vi "main(Test DQMH modules).bak.vi"() -> ()   [LabVIEW 2018, in "Application.lvlib"] (continued)
            n2019 = Select(t="Quece timeout", s=w4663, f=w4660) -> (s? t:f=w4659:string)
            n2020 = call "string log (SubVI).vi"("Enum"=enum16{"Init", "Log", "Read"}."Log", "state Name"=w4659) -> ()  [unwired: 8 in, 2 out]
          }
          frame condition #1 {
          }
        }
        n2021 = call "progress string(SubVI).vi"("String 3"=w4625, "String in"=w4626) -> ("String out"=w4627:string)  [unwired: 9 in]
        n2022 = call "FGV Driver Data.vi"("DUT index(1-60)"=w4624) -> ("DUT SC"=w4623:bool)  [unwired: 7 in, 3 out]
        n2023 = case shown="False" w4623 {
          tunnel: [w4652 _] -> w4632
          tunnel: w4629 -> [w4651 _]
          frame False {
            w4639 = T11 {"command"="", "command data"=variant} ("element")
            w4638 = "MEAS.mux6_1"
            n2024 = To Variant(anything=T4."mux6-1_channel0" ("mux6_1(3wires)_encode")) -> (Variant=w4637:variant)
            n2025 = To Variant(anything=T4."mux6_1_channel5_3" ("mux6_1(3wires)_encode")) -> (Variant=w4649:variant)
            n2026 = To Variant(anything=T4."mux6_1_channel5_2" ("mux6_1(3wires)_encode")) -> (Variant=w4647:variant)
            n2027 = Bundle By Name(cluster=w4639, "command"=w4638, "command data"=w4647) -> (w4646:T11)
            n2028 = Bundle By Name(cluster=w4639, "command"=w4638, "command data"=w4649) -> (w4645:T11)
            n2029 = Bundle By Name(cluster=w4639, "command"=w4638, "command data"=w4637) -> ()  [unwired: 1 out]
            n2030 = Bundle By Name(cluster=w4639, "command"="MEAS.DMM dual read") -> (w4643:T11)
            n2031 = Build Array(w4646, w4645, w4643) -> (w4641:T11[])
            n2032 = Reverse 1D Array(array=w4641) -> (reversed array=w4642:T11[])
            n2033 = for {
              tunnel: [w4658] -> w4652 mode=indexing
              tunnel: w4651 -> [w4657]
              tunnel: w4642 -> [w4656] mode=indexing
              n2034 = Unbundle By Name(w4656) -> ("command"=w4655:string, "command data"=w4654:variant)
              n2035 = call "App enquece.vi"("Priority Enquece"=TRUE, "command data"=w4654, "command"=w4655, "queue in"=w4657) -> ("error out"=w4658:errorcluster)  [unwired: 6 in, 1 out]
            }
          }
          frame True {
          }
        }
        n2036 = Merge Errors(w4630, w4632) -> (w4631:errorcluster)
      }
      frame "Test DRV 36" {
        w4665 = 36  # DUT index(0-59)
        n2037 = disable-structure shown="LOGGING==TRUE" {
          disable-tunnel: w4666 -> [w4701 _]
          frame condition #0 (active) {
            n2038 = Empty String/Path?(string/path=w4701) -> (empty?=w4704:bool)
            n2039 = Select(t="Quece timeout", s=w4704, f=w4701) -> (s? t:f=w4700:string)
            n2040 = call "string log (SubVI).vi"("Enum"=enum16{"Init", "Log", "Read"}."Log", "state Name"=w4700) -> ()  [unwired: 8 in, 2 out]
          }
          frame condition #1 {
          }
        }
        n2041 = call "progress string(SubVI).vi"("String 3"=w4666, "String in"=w4667) -> ("String out"=w4668:string)  [unwired: 9 in]
        n2042 = call "FGV Driver Data.vi"("DUT index(1-60)"=w4665) -> ("DUT SC"=w4664:bool)  [unwired: 7 in, 3 out]
        n2043 = case shown="False" w4664 {
          tunnel: [w4693 _] -> w4673
          tunnel: w4670 -> [w4692 _]
          frame False {
            w4680 = T11 {"command"="", "command data"=variant} ("element")
            w4679 = "MEAS.mux6_1"
            n2044 = To Variant(anything=T4."mux6-1_channel0" ("mux6_1(3wires)_encode")) -> (Variant=w4678:variant)
            n2045 = To Variant(anything=T4."mux6_1_channel6_3" ("mux6_1(3wires)_encode")) -> (Variant=w4690:variant)
            n2046 = To Variant(anything=T4."mux6_1_channel6_2" ("mux6_1(3wires)_encode")) -> (Variant=w4688:variant)
            n2047 = Bundle By Name(cluster=w4680, "command"=w4679, "command data"=w4688) -> (w4687:T11)
            n2048 = Bundle By Name(cluster=w4680, "command"=w4679, "command data"=w4690) -> (w4686:T11)
            n2049 = Bundle By Name(cluster=w4680, "command"=w4679, "command data"=w4678) -> ()  [unwired: 1 out]
            n2050 = Bundle By Name(cluster=w4680, "command"="MEAS.DMM dual read") -> (w4684:T11)
            n2051 = Build Array(w4687, w4686, w4684) -> (w4682:T11[])
            n2052 = Reverse 1D Array(array=w4682) -> (reversed array=w4683:T11[])
            n2053 = for {
              tunnel: [w4699] -> w4693 mode=indexing
              tunnel: w4692 -> [w4698]
              tunnel: w4683 -> [w4697] mode=indexing
              n2054 = Unbundle By Name(w4697) -> ("command"=w4696:string, "command data"=w4695:variant)
              n2055 = call "App enquece.vi"("Priority Enquece"=TRUE, "command data"=w4695, "command"=w4696, "queue in"=w4698) -> ("error out"=w4699:errorcluster)  [unwired: 6 in, 1 out]
            }
          }
          frame True {
          }
        }
        n2056 = Merge Errors(w4671, w4673) -> (w4672:errorcluster)
      }
      frame "Test DRV 37" {
        w4706 = 37  # DUT index(0-59)
        n2057 = disable-structure shown="LOGGING==TRUE" {
          disable-tunnel: w4707 -> [w4742 _]
          frame condition #0 (active) {
            n2058 = Empty String/Path?(string/path=w4742) -> (empty?=w4745:bool)
            n2059 = Select(t="Quece timeout", s=w4745, f=w4742) -> (s? t:f=w4741:string)
            n2060 = call "string log (SubVI).vi"("Enum"=enum16{"Init", "Log", "Read"}."Log", "state Name"=w4741) -> ()  [unwired: 8 in, 2 out]
          }
          frame condition #1 {
          }
        }
        n2061 = call "progress string(SubVI).vi"("String 3"=w4707, "String in"=w4708) -> ("String out"=w4709:string)  [unwired: 9 in]
        n2062 = call "FGV Driver Data.vi"("DUT index(1-60)"=w4706) -> ("DUT SC"=w4705:bool)  [unwired: 7 in, 3 out]
        n2063 = case shown="False" w4705 {
          tunnel: [w4734 _] -> w4714
          tunnel: w4711 -> [w4733 _]
          frame False {
            w4721 = T11 {"command"="", "command data"=variant} ("element")
            w4720 = "MEAS.mux6_1"
            n2064 = To Variant(anything=T4."mux6-1_channel0" ("mux6_1(3wires)_encode")) -> (Variant=w4719:variant)
            n2065 = To Variant(anything=T4."mux6_1_channel1_3" ("mux6_1(3wires)_encode")) -> (Variant=w4731:variant)
            n2066 = To Variant(anything=T4."mux6-1_channel1_2" ("mux6_1(3wires)_encode")) -> (Variant=w4729:variant)
            n2067 = Bundle By Name(cluster=w4721, "command"=w4720, "command data"=w4729) -> (w4728:T11)
            n2068 = Bundle By Name(cluster=w4721, "command"=w4720, "command data"=w4731) -> (w4727:T11)
            n2069 = Bundle By Name(cluster=w4721, "command"=w4720, "command data"=w4719) -> ()  [unwired: 1 out]
            n2070 = Bundle By Name(cluster=w4721, "command"="MEAS.DMM dual read") -> (w4725:T11)
            n2071 = Build Array(w4728, w4727, w4725) -> (w4723:T11[])
            n2072 = Reverse 1D Array(array=w4723) -> (reversed array=w4724:T11[])
            n2073 = for {
              tunnel: [w4740] -> w4734 mode=indexing
              tunnel: w4733 -> [w4739]
              tunnel: w4724 -> [w4738] mode=indexing
              n2074 = Unbundle By Name(w4738) -> ("command"=w4737:string, "command data"=w4736:variant)
              n2075 = call "App enquece.vi"("Priority Enquece"=TRUE, "command data"=w4736, "command"=w4737, "queue in"=w4739) -> ("error out"=w4740:errorcluster)  [unwired: 6 in, 1 out]
            }
          }
          frame True {
          }
        }
        n2076 = Merge Errors(w4712, w4714) -> (w4713:errorcluster)
      }
      frame "Test DRV 38" {
        w4747 = 38  # DUT index(0-59)
        n2077 = disable-structure shown="LOGGING==TRUE" {
          disable-tunnel: w4748 -> [w4783 _]
          frame condition #0 (active) {
            n2078 = Empty String/Path?(string/path=w4783) -> (empty?=w4786:bool)
            n2079 = Select(t="Quece timeout", s=w4786, f=w4783) -> (s? t:f=w4782:string)
            n2080 = call "string log (SubVI).vi"("Enum"=enum16{"Init", "Log", "Read"}."Log", "state Name"=w4782) -> ()  [unwired: 8 in, 2 out]
          }
          frame condition #1 {
          }
        }
        n2081 = call "progress string(SubVI).vi"("String 3"=w4748, "String in"=w4749) -> ("String out"=w4750:string)  [unwired: 9 in]
        n2082 = call "FGV Driver Data.vi"("DUT index(1-60)"=w4747) -> ("DUT SC"=w4746:bool)  [unwired: 7 in, 3 out]
        n2083 = case shown="False" w4746 {
          tunnel: [w4775 _] -> w4755
          tunnel: w4752 -> [w4774 _]
          frame False {
            w4762 = T11 {"command"="", "command data"=variant} ("element")
            w4761 = "MEAS.mux6_1"
            n2084 = To Variant(anything=T4."mux6-1_channel0" ("mux6_1(3wires)_encode")) -> (Variant=w4760:variant)
            n2085 = To Variant(anything=T4."mux6_1_channel2_3" ("mux6_1(3wires)_encode")) -> (Variant=w4772:variant)
            n2086 = To Variant(anything=T4."mux6_1_channel2_2" ("mux6_1(3wires)_encode")) -> (Variant=w4770:variant)
            n2087 = Bundle By Name(cluster=w4762, "command"=w4761, "command data"=w4770) -> (w4769:T11)
            n2088 = Bundle By Name(cluster=w4762, "command"=w4761, "command data"=w4772) -> (w4768:T11)
            n2089 = Bundle By Name(cluster=w4762, "command"=w4761, "command data"=w4760) -> ()  [unwired: 1 out]
            n2090 = Bundle By Name(cluster=w4762, "command"="MEAS.DMM dual read") -> (w4766:T11)
            n2091 = Build Array(w4769, w4768, w4766) -> (w4764:T11[])
            n2092 = Reverse 1D Array(array=w4764) -> (reversed array=w4765:T11[])
            n2093 = for {
              tunnel: [w4781] -> w4775 mode=indexing
              tunnel: w4774 -> [w4780]
              tunnel: w4765 -> [w4779] mode=indexing
              n2094 = Unbundle By Name(w4779) -> ("command"=w4778:string, "command data"=w4777:variant)
              n2095 = call "App enquece.vi"("Priority Enquece"=TRUE, "command data"=w4777, "command"=w4778, "queue in"=w4780) -> ("error out"=w4781:errorcluster)  [unwired: 6 in, 1 out]
            }
          }
          frame True {
          }
        }
        n2096 = Merge Errors(w4753, w4755) -> (w4754:errorcluster)
      }
      frame "Test DRV 39" {
        w4787 = 39  # DUT index(0-59)
        n2097 = disable-structure shown="LOGGING==TRUE" {
          disable-tunnel: w4789 -> [w4824 _]
          frame condition #0 (active) {
            n2098 = Empty String/Path?(string/path=w4824) -> (empty?=w4827:bool)
            n2099 = Select(t="Quece timeout", s=w4827, f=w4824) -> (s? t:f=w4823:string)
            n2100 = call "string log (SubVI).vi"("Enum"=enum16{"Init", "Log", "Read"}."Log", "state Name"=w4823) -> ()  [unwired: 8 in, 2 out]
          }
          frame condition #1 {
          }
        }
        n2101 = call "progress string(SubVI).vi"("String 3"=w4789, "String in"=w4790) -> ("String out"=w4791:string)  [unwired: 9 in]
        n2102 = call "FGV Driver Data.vi"("DUT index(1-60)"=w4787) -> ("DUT SC"=w4788:bool)  [unwired: 7 in, 3 out]
        n2103 = case shown="False" w4788 {
          tunnel: [w4816 _] -> w4796
          tunnel: w4793 -> [w4815 _]
          frame False {
            w4803 = T11 {"command"="", "command data"=variant} ("element")
            w4802 = "MEAS.mux6_1"
            n2104 = To Variant(anything=T4."mux6-1_channel0" ("mux6_1(3wires)_encode")) -> (Variant=w4801:variant)
            n2105 = To Variant(anything=T4."mux6_1_channel3_3" ("mux6_1(3wires)_encode")) -> (Variant=w4813:variant)
            n2106 = To Variant(anything=T4."mux6_1_channel3_2" ("mux6_1(3wires)_encode")) -> (Variant=w4811:variant)
            n2107 = Bundle By Name(cluster=w4803, "command"=w4802, "command data"=w4811) -> (w4810:T11)
            n2108 = Bundle By Name(cluster=w4803, "command"=w4802, "command data"=w4813) -> (w4809:T11)
            n2109 = Bundle By Name(cluster=w4803, "command"=w4802, "command data"=w4801) -> ()  [unwired: 1 out]
            n2110 = Bundle By Name(cluster=w4803, "command"="MEAS.DMM dual read") -> (w4807:T11)
            n2111 = Build Array(w4810, w4809, w4807) -> (w4805:T11[])
            n2112 = Reverse 1D Array(array=w4805) -> (reversed array=w4806:T11[])
            n2113 = for {
              tunnel: [w4822] -> w4816 mode=indexing
              tunnel: w4815 -> [w4821]
              tunnel: w4806 -> [w4820] mode=indexing
              n2114 = Unbundle By Name(w4820) -> ("command"=w4819:string, "command data"=w4818:variant)
              n2115 = call "App enquece.vi"("Priority Enquece"=TRUE, "command data"=w4818, "command"=w4819, "queue in"=w4821) -> ("error out"=w4822:errorcluster)  [unwired: 6 in, 1 out]
            }
          }
          frame True {
          }
        }
        n2116 = Merge Errors(w4794, w4796) -> (w4795:errorcluster)
      }
      frame "Test DRV 40" {
        w4829 = 40  # DUT index(0-59)
        n2117 = disable-structure shown="LOGGING==TRUE" {
          disable-tunnel: w4830 -> [w4865 _]
          frame condition #0 (active) {
            n2118 = Empty String/Path?(string/path=w4865) -> (empty?=w4868:bool)
            n2119 = Select(t="Quece timeout", s=w4868, f=w4865) -> (s? t:f=w4864:string)
            n2120 = call "string log (SubVI).vi"("Enum"=enum16{"Init", "Log", "Read"}."Log", "state Name"=w4864) -> ()  [unwired: 8 in, 2 out]
          }
          frame condition #1 {
          }
        }
        n2121 = call "progress string(SubVI).vi"("String 3"=w4830, "String in"=w4831) -> ("String out"=w4832:string)  [unwired: 9 in]
        n2122 = call "FGV Driver Data.vi"("DUT index(1-60)"=w4829) -> ("DUT SC"=w4828:bool)  [unwired: 7 in, 3 out]
        n2123 = case shown="False" w4828 {
          tunnel: [w4857 _] -> w4837
          tunnel: w4834 -> [w4856 _]
          frame False {
            w4844 = T11 {"command"="", "command data"=variant} ("element")
            w4843 = "MEAS.mux6_1"
            n2124 = To Variant(anything=T4."mux6-1_channel0" ("mux6_1(3wires)_encode")) -> (Variant=w4842:variant)
            n2125 = To Variant(anything=T4."mux6_1_channel4_3" ("mux6_1(3wires)_encode")) -> (Variant=w4854:variant)
            n2126 = To Variant(anything=T4."mux6_1_channel4_2" ("mux6_1(3wires)_encode")) -> (Variant=w4852:variant)
            n2127 = Bundle By Name(cluster=w4844, "command"=w4843, "command data"=w4852) -> (w4851:T11)
            n2128 = Bundle By Name(cluster=w4844, "command"=w4843, "command data"=w4854) -> (w4850:T11)
            n2129 = Bundle By Name(cluster=w4844, "command"=w4843, "command data"=w4842) -> ()  [unwired: 1 out]
            n2130 = Bundle By Name(cluster=w4844, "command"="MEAS.DMM dual read") -> (w4848:T11)
            n2131 = Build Array(w4851, w4850, w4848) -> (w4846:T11[])
            n2132 = Reverse 1D Array(array=w4846) -> (reversed array=w4847:T11[])
            n2133 = for {
              tunnel: [w4863] -> w4857 mode=indexing
              tunnel: w4856 -> [w4862]
              tunnel: w4847 -> [w4861] mode=indexing
              n2134 = Unbundle By Name(w4861) -> ("command"=w4860:string, "command data"=w4859:variant)
              n2135 = call "App enquece.vi"("Priority Enquece"=TRUE, "command data"=w4859, "command"=w4860, "queue in"=w4862) -> ("error out"=w4863:errorcluster)  [unwired: 6 in, 1 out]
            }
          }
          frame True {
          }
        }
        n2136 = Merge Errors(w4835, w4837) -> (w4836:errorcluster)
      }
      frame "Test DRV 41" {
        w4870 = 41  # DUT index(0-59)
        n2137 = disable-structure shown="LOGGING==TRUE" {
          disable-tunnel: w4871 -> [w4906 _]
          frame condition #0 (active) {
            n2138 = Empty String/Path?(string/path=w4906) -> (empty?=w4909:bool)
            n2139 = Select(t="Quece timeout", s=w4909, f=w4906) -> (s? t:f=w4905:string)
            n2140 = call "string log (SubVI).vi"("Enum"=enum16{"Init", "Log", "Read"}."Log", "state Name"=w4905) -> ()  [unwired: 8 in, 2 out]
          }
          frame condition #1 {
          }
        }
        n2141 = call "progress string(SubVI).vi"("String 3"=w4871, "String in"=w4872) -> ("String out"=w4873:string)  [unwired: 9 in]
        n2142 = call "FGV Driver Data.vi"("DUT index(1-60)"=w4870) -> ("DUT SC"=w4869:bool)  [unwired: 7 in, 3 out]
        n2143 = case shown="False" w4869 {
          tunnel: [w4898 _] -> w4878
          tunnel: w4875 -> [w4897 _]
          frame False {
            w4885 = T11 {"command"="", "command data"=variant} ("element")
            w4884 = "MEAS.mux6_1"
            n2144 = To Variant(anything=T4."mux6-1_channel0" ("mux6_1(3wires)_encode")) -> (Variant=w4883:variant)
            n2145 = To Variant(anything=T4."mux6_1_channel5_3" ("mux6_1(3wires)_encode")) -> (Variant=w4895:variant)
            n2146 = To Variant(anything=T4."mux6_1_channel5_2" ("mux6_1(3wires)_encode")) -> (Variant=w4893:variant)
            n2147 = Bundle By Name(cluster=w4885, "command"=w4884, "command data"=w4893) -> (w4892:T11)
            n2148 = Bundle By Name(cluster=w4885, "command"=w4884, "command data"=w4895) -> (w4891:T11)
            n2149 = Bundle By Name(cluster=w4885, "command"=w4884, "command data"=w4883) -> ()  [unwired: 1 out]
            n2150 = Bundle By Name(cluster=w4885, "command"="MEAS.DMM dual read") -> (w4889:T11)
            n2151 = Build Array(w4892, w4891, w4889) -> (w4887:T11[])
            n2152 = Reverse 1D Array(array=w4887) -> (reversed array=w4888:T11[])
            n2153 = for {
              tunnel: [w4904] -> w4898 mode=indexing
              tunnel: w4897 -> [w4903]
              tunnel: w4888 -> [w4902] mode=indexing
              n2154 = Unbundle By Name(w4902) -> ("command"=w4901:string, "command data"=w4900:variant)
              n2155 = call "App enquece.vi"("Priority Enquece"=TRUE, "command data"=w4900, "command"=w4901, "queue in"=w4903) -> ("error out"=w4904:errorcluster)  [unwired: 6 in, 1 out]
            }
          }
          frame True {
          }
        }
        n2156 = Merge Errors(w4876, w4878) -> (w4877:errorcluster)
      }
      frame "Test DRV 42" {
        w4911 = 42  # DUT index(0-59)
        n2157 = disable-structure shown="LOGGING==TRUE" {
          disable-tunnel: w4912 -> [w4947 _]
          frame condition #0 (active) {
            n2158 = Empty String/Path?(string/path=w4947) -> (empty?=w4950:bool)
            n2159 = Select(t="Quece timeout", s=w4950, f=w4947) -> (s? t:f=w4946:string)
            n2160 = call "string log (SubVI).vi"("Enum"=enum16{"Init", "Log", "Read"}."Log", "state Name"=w4946) -> ()  [unwired: 8 in, 2 out]
          }
          frame condition #1 {
          }
        }
        n2161 = call "progress string(SubVI).vi"("String 3"=w4912, "String in"=w4913) -> ("String out"=w4914:string)  [unwired: 9 in]
        n2162 = call "FGV Driver Data.vi"("DUT index(1-60)"=w4911) -> ("DUT SC"=w4910:bool)  [unwired: 7 in, 3 out]
        n2163 = case shown="False" w4910 {
          tunnel: [w4939 _] -> w4919
          tunnel: w4916 -> [w4938 _]
          frame False {
            w4926 = T11 {"command"="", "command data"=variant} ("element")
            w4925 = "MEAS.mux6_1"
            n2164 = To Variant(anything=T4."mux6-1_channel0" ("mux6_1(3wires)_encode")) -> (Variant=w4924:variant)
            n2165 = To Variant(anything=T4."mux6_1_channel6_3" ("mux6_1(3wires)_encode")) -> (Variant=w4936:variant)
            n2166 = To Variant(anything=T4."mux6_1_channel6_2" ("mux6_1(3wires)_encode")) -> (Variant=w4934:variant)
            n2167 = Bundle By Name(cluster=w4926, "command"=w4925, "command data"=w4934) -> (w4933:T11)
            n2168 = Bundle By Name(cluster=w4926, "command"=w4925, "command data"=w4936) -> (w4932:T11)
            n2169 = Bundle By Name(cluster=w4926, "command"=w4925, "command data"=w4924) -> ()  [unwired: 1 out]
            n2170 = Bundle By Name(cluster=w4926, "command"="MEAS.DMM dual read") -> (w4930:T11)
            n2171 = Build Array(w4933, w4932, w4930) -> (w4928:T11[])
            n2172 = Reverse 1D Array(array=w4928) -> (reversed array=w4929:T11[])
            n2173 = for {
              tunnel: [w4945] -> w4939 mode=indexing
              tunnel: w4938 -> [w4944]
              tunnel: w4929 -> [w4943] mode=indexing
              n2174 = Unbundle By Name(w4943) -> ("command"=w4942:string, "command data"=w4941:variant)
              n2175 = call "App enquece.vi"("Priority Enquece"=TRUE, "command data"=w4941, "command"=w4942, "queue in"=w4944) -> ("error out"=w4945:errorcluster)  [unwired: 6 in, 1 out]
            }
          }
          frame True {
          }
        }
        n2176 = Merge Errors(w4917, w4919) -> (w4918:errorcluster)
      }
      frame "Test DRV 43" {
        w4952 = 43  # DUT index(0-59)
        n2177 = disable-structure shown="LOGGING==TRUE" {
          disable-tunnel: w4953 -> [w4988 _]
          frame condition #0 (active) {
            n2178 = Empty String/Path?(string/path=w4988) -> (empty?=w4991:bool)
            n2179 = Select(t="Quece timeout", s=w4991, f=w4988) -> (s? t:f=w4987:string)
            n2180 = call "string log (SubVI).vi"("Enum"=enum16{"Init", "Log", "Read"}."Log", "state Name"=w4987) -> ()  [unwired: 8 in, 2 out]
          }
          frame condition #1 {
          }
        }
        n2181 = call "progress string(SubVI).vi"("String 3"=w4953, "String in"=w4954) -> ("String out"=w4955:string)  [unwired: 9 in]
        n2182 = call "FGV Driver Data.vi"("DUT index(1-60)"=w4952) -> ("DUT SC"=w4951:bool)  [unwired: 7 in, 3 out]
        n2183 = case shown="False" w4951 {
          tunnel: [w4980 _] -> w4960
          tunnel: w4957 -> [w4979 _]
          frame False {
            w4967 = T11 {"command"="", "command data"=variant} ("element")
            w4966 = "MEAS.mux6_1"
            n2184 = To Variant(anything=T4."mux6-1_channel0" ("mux6_1(3wires)_encode")) -> (Variant=w4965:variant)
            n2185 = To Variant(anything=T4."mux6_1_channel1_3" ("mux6_1(3wires)_encode")) -> (Variant=w4977:variant)
            n2186 = To Variant(anything=T4."mux6-1_channel1_2" ("mux6_1(3wires)_encode")) -> (Variant=w4975:variant)
            n2187 = Bundle By Name(cluster=w4967, "command"=w4966, "command data"=w4975) -> (w4974:T11)
            n2188 = Bundle By Name(cluster=w4967, "command"=w4966, "command data"=w4977) -> (w4973:T11)
            n2189 = Bundle By Name(cluster=w4967, "command"=w4966, "command data"=w4965) -> ()  [unwired: 1 out]
            n2190 = Bundle By Name(cluster=w4967, "command"="MEAS.DMM dual read") -> (w4971:T11)
            n2191 = Build Array(w4974, w4973, w4971) -> (w4969:T11[])
            n2192 = Reverse 1D Array(array=w4969) -> (reversed array=w4970:T11[])
            n2193 = for {
              tunnel: [w4986] -> w4980 mode=indexing
              tunnel: w4979 -> [w4985]
              tunnel: w4970 -> [w4984] mode=indexing
              n2194 = Unbundle By Name(w4984) -> ("command"=w4983:string, "command data"=w4982:variant)
              n2195 = call "App enquece.vi"("Priority Enquece"=TRUE, "command data"=w4982, "command"=w4983, "queue in"=w4985) -> ("error out"=w4986:errorcluster)  [unwired: 6 in, 1 out]
            }
          }
          frame True {
          }
        }
        n2196 = Merge Errors(w4958, w4960) -> (w4959:errorcluster)
      }
      frame "Test DRV 44" {
        w4993 = 44  # DUT index(0-59)
        n2197 = disable-structure shown="LOGGING==TRUE" {
          disable-tunnel: w4994 -> [w5029 _]
          frame condition #0 (active) {
            n2198 = Empty String/Path?(string/path=w5029) -> (empty?=w5032:bool)
            n2199 = Select(t="Quece timeout", s=w5032, f=w5029) -> (s? t:f=w5028:string)
            n2200 = call "string log (SubVI).vi"("Enum"=enum16{"Init", "Log", "Read"}."Log", "state Name"=w5028) -> ()  [unwired: 8 in, 2 out]
          }
          frame condition #1 {
          }
        }
        n2201 = call "progress string(SubVI).vi"("String 3"=w4994, "String in"=w4995) -> ("String out"=w4996:string)  [unwired: 9 in]
        n2202 = call "FGV Driver Data.vi"("DUT index(1-60)"=w4993) -> ("DUT SC"=w4992:bool)  [unwired: 7 in, 3 out]
        n2203 = case shown="False" w4992 {
          tunnel: [w5021 _] -> w5001
          tunnel: w4998 -> [w5020 _]
          frame False {
            w5008 = T11 {"command"="", "command data"=variant} ("element")
            w5007 = "MEAS.mux6_1"
            n2204 = To Variant(anything=T4."mux6-1_channel0" ("mux6_1(3wires)_encode")) -> (Variant=w5006:variant)
            n2205 = To Variant(anything=T4."mux6_1_channel2_3" ("mux6_1(3wires)_encode")) -> (Variant=w5018:variant)
            n2206 = To Variant(anything=T4."mux6_1_channel2_2" ("mux6_1(3wires)_encode")) -> (Variant=w5016:variant)
            n2207 = Bundle By Name(cluster=w5008, "command"=w5007, "command data"=w5016) -> (w5015:T11)
            n2208 = Bundle By Name(cluster=w5008, "command"=w5007, "command data"=w5018) -> (w5014:T11)
            n2209 = Bundle By Name(cluster=w5008, "command"=w5007, "command data"=w5006) -> ()  [unwired: 1 out]
            n2210 = Bundle By Name(cluster=w5008, "command"="MEAS.DMM dual read") -> (w5012:T11)
            n2211 = Build Array(w5015, w5014, w5012) -> (w5010:T11[])
            n2212 = Reverse 1D Array(array=w5010) -> (reversed array=w5011:T11[])
            n2213 = for {
              tunnel: [w5027] -> w5021 mode=indexing
              tunnel: w5020 -> [w5026]
              tunnel: w5011 -> [w5025] mode=indexing
              n2214 = Unbundle By Name(w5025) -> ("command"=w5024:string, "command data"=w5023:variant)
              n2215 = call "App enquece.vi"("Priority Enquece"=TRUE, "command data"=w5023, "command"=w5024, "queue in"=w5026) -> ("error out"=w5027:errorcluster)  [unwired: 6 in, 1 out]
            }
          }
          frame True {
          }
        }
        n2216 = Merge Errors(w4999, w5001) -> (w5000:errorcluster)
      }
      frame "Test DRV 45" {
        w5033 = 45  # DUT index(1-60)
        n2217 = disable-structure shown="LOGGING==TRUE" {
          disable-tunnel: w5035 -> [w5070 _]
          frame condition #0 (active) {
            n2218 = Empty String/Path?(string/path=w5070) -> (empty?=w5073:bool)
            n2219 = Select(t="Quece timeout", s=w5073, f=w5070) -> (s? t:f=w5069:string)
            n2220 = call "string log (SubVI).vi"("Enum"=enum16{"Init", "Log", "Read"}."Log", "state Name"=w5069) -> ()  [unwired: 8 in, 2 out]
          }
          frame condition #1 {
          }
        }
        n2221 = call "progress string(SubVI).vi"("String 3"=w5035, "String in"=w5036) -> ("String out"=w5037:string)  [unwired: 9 in]
        n2222 = call "FGV Driver Data.vi"("DUT index(1-60)"=w5033) -> ("DUT SC"=w5034:bool)  [unwired: 7 in, 3 out]
        n2223 = case shown="False" w5034 {
          tunnel: [w5062 _] -> w5042
          tunnel: w5039 -> [w5061 _]
          frame False {
            w5049 = T11 {"command"="", "command data"=variant} ("element")
            w5048 = "MEAS.mux6_1"
            n2224 = To Variant(anything=T4."mux6-1_channel0" ("mux6_1(3wires)_encode")) -> (Variant=w5047:variant)
            n2225 = To Variant(anything=T4."mux6_1_channel3_3" ("mux6_1(3wires)_encode")) -> (Variant=w5059:variant)
            n2226 = To Variant(anything=T4."mux6_1_channel3_2" ("mux6_1(3wires)_encode")) -> (Variant=w5057:variant)
            n2227 = Bundle By Name(cluster=w5049, "command"=w5048, "command data"=w5057) -> (w5056:T11)
            n2228 = Bundle By Name(cluster=w5049, "command"=w5048, "command data"=w5059) -> (w5055:T11)
            n2229 = Bundle By Name(cluster=w5049, "command"=w5048, "command data"=w5047) -> ()  [unwired: 1 out]
            n2230 = Bundle By Name(cluster=w5049, "command"="MEAS.DMM dual read") -> (w5053:T11)
            n2231 = Build Array(w5056, w5055, w5053) -> (w5051:T11[])
            n2232 = Reverse 1D Array(array=w5051) -> (reversed array=w5052:T11[])
            n2233 = for {
              tunnel: [w5068] -> w5062 mode=indexing
              tunnel: w5061 -> [w5067]
              tunnel: w5052 -> [w5066] mode=indexing
              n2234 = Unbundle By Name(w5066) -> ("command"=w5065:string, "command data"=w5064:variant)
              n2235 = call "App enquece.vi"("Priority Enquece"=TRUE, "command data"=w5064, "command"=w5065, "queue in"=w5067) -> ("error out"=w5068:errorcluster)  [unwired: 6 in, 1 out]
            }
          }
          frame True {
          }
        }
        n2236 = Merge Errors(w5040, w5042) -> (w5041:errorcluster)
      }
      frame "Test DRV 46" {
        w5075 = 46  # DUT index(0-59)
        n2237 = disable-structure shown="LOGGING==TRUE" {
          disable-tunnel: w5076 -> [w5111 _]
          frame condition #0 (active) {
            n2238 = Empty String/Path?(string/path=w5111) -> (empty?=w5114:bool)
            n2239 = Select(t="Quece timeout", s=w5114, f=w5111) -> (s? t:f=w5110:string)
            n2240 = call "string log (SubVI).vi"("Enum"=enum16{"Init", "Log", "Read"}."Log", "state Name"=w5110) -> ()  [unwired: 8 in, 2 out]
          }
          frame condition #1 {
          }
        }
        n2241 = call "progress string(SubVI).vi"("String 3"=w5076, "String in"=w5077) -> ("String out"=w5078:string)  [unwired: 9 in]
        n2242 = call "FGV Driver Data.vi"("DUT index(1-60)"=w5075) -> ("DUT SC"=w5074:bool)  [unwired: 7 in, 3 out]
        n2243 = case shown="False" w5074 {
          tunnel: [w5103 _] -> w5083
          tunnel: w5080 -> [w5102 _]
          frame False {
            w5090 = T11 {"command"="", "command data"=variant} ("element")
            w5089 = "MEAS.mux6_1"
            n2244 = To Variant(anything=T4."mux6-1_channel0" ("mux6_1(3wires)_encode")) -> (Variant=w5088:variant)
            n2245 = To Variant(anything=T4."mux6_1_channel4_3" ("mux6_1(3wires)_encode")) -> (Variant=w5100:variant)
            n2246 = To Variant(anything=T4."mux6_1_channel4_2" ("mux6_1(3wires)_encode")) -> (Variant=w5098:variant)
            n2247 = Bundle By Name(cluster=w5090, "command"=w5089, "command data"=w5098) -> (w5097:T11)
            n2248 = Bundle By Name(cluster=w5090, "command"=w5089, "command data"=w5100) -> (w5096:T11)
            n2249 = Bundle By Name(cluster=w5090, "command"=w5089, "command data"=w5088) -> ()  [unwired: 1 out]
            n2250 = Bundle By Name(cluster=w5090, "command"="MEAS.DMM dual read") -> (w5094:T11)
            n2251 = Build Array(w5097, w5096, w5094) -> (w5092:T11[])
            n2252 = Reverse 1D Array(array=w5092) -> (reversed array=w5093:T11[])
            n2253 = for {
              tunnel: [w5109] -> w5103 mode=indexing
              tunnel: w5102 -> [w5108]
              tunnel: w5093 -> [w5107] mode=indexing
              n2254 = Unbundle By Name(w5107) -> ("command"=w5106:string, "command data"=w5105:variant)
              n2255 = call "App enquece.vi"("Priority Enquece"=TRUE, "command data"=w5105, "command"=w5106, "queue in"=w5108) -> ("error out"=w5109:errorcluster)  [unwired: 6 in, 1 out]
            }
          }
          frame True {
          }
        }
        n2256 = Merge Errors(w5081, w5083) -> (w5082:errorcluster)
      }
      frame "Test DRV 47" {
        w5115 = 47  # DUT index(0-59)
        n2257 = disable-structure shown="LOGGING==TRUE" {
          disable-tunnel: w5117 -> [w5152 _]
          frame condition #0 (active) {
            n2258 = Empty String/Path?(string/path=w5152) -> (empty?=w5155:bool)
            n2259 = Select(t="Quece timeout", s=w5155, f=w5152) -> (s? t:f=w5151:string)
            n2260 = call "string log (SubVI).vi"("Enum"=enum16{"Init", "Log", "Read"}."Log", "state Name"=w5151) -> ()  [unwired: 8 in, 2 out]
          }
          frame condition #1 {
          }
        }
        n2261 = call "progress string(SubVI).vi"("String 3"=w5117, "String in"=w5118) -> ("String out"=w5119:string)  [unwired: 9 in]
        n2262 = call "FGV Driver Data.vi"("DUT index(1-60)"=w5115) -> ("DUT SC"=w5116:bool)  [unwired: 7 in, 3 out]
        n2263 = case shown="False" w5116 {
          tunnel: [w5144 _] -> w5124
          tunnel: w5121 -> [w5143 _]
          frame False {
            w5131 = T11 {"command"="", "command data"=variant} ("element")
            w5130 = "MEAS.mux6_1"
            n2264 = To Variant(anything=T4."mux6-1_channel0" ("mux6_1(3wires)_encode")) -> (Variant=w5129:variant)
            n2265 = To Variant(anything=T4."mux6_1_channel5_3" ("mux6_1(3wires)_encode")) -> (Variant=w5141:variant)
            n2266 = To Variant(anything=T4."mux6_1_channel5_2" ("mux6_1(3wires)_encode")) -> (Variant=w5139:variant)
            n2267 = Bundle By Name(cluster=w5131, "command"=w5130, "command data"=w5139) -> (w5138:T11)
            n2268 = Bundle By Name(cluster=w5131, "command"=w5130, "command data"=w5141) -> (w5137:T11)
            n2269 = Bundle By Name(cluster=w5131, "command"=w5130, "command data"=w5129) -> ()  [unwired: 1 out]
            n2270 = Bundle By Name(cluster=w5131, "command"="MEAS.DMM dual read") -> (w5135:T11)
            n2271 = Build Array(w5138, w5137, w5135) -> (w5133:T11[])
            n2272 = Reverse 1D Array(array=w5133) -> (reversed array=w5134:T11[])
            n2273 = for {
              tunnel: [w5150] -> w5144 mode=indexing
              tunnel: w5143 -> [w5149]
              tunnel: w5134 -> [w5148] mode=indexing
              n2274 = Unbundle By Name(w5148) -> ("command"=w5147:string, "command data"=w5146:variant)
              n2275 = call "App enquece.vi"("Priority Enquece"=TRUE, "command data"=w5146, "command"=w5147, "queue in"=w5149) -> ("error out"=w5150:errorcluster)  [unwired: 6 in, 1 out]
            }
          }
          frame True {
          }
        }
        n2276 = Merge Errors(w5122, w5124) -> (w5123:errorcluster)
      }
      frame "Test DRV 48" {
        w5157 = 48  # DUT index(0-59)
        n2277 = disable-structure shown="LOGGING==TRUE" {
          disable-tunnel: w5158 -> [w5193 _]
          frame condition #0 (active) {
            n2278 = Empty String/Path?(string/path=w5193) -> (empty?=w5196:bool)
            n2279 = Select(t="Quece timeout", s=w5196, f=w5193) -> (s? t:f=w5192:string)
            n2280 = call "string log (SubVI).vi"("Enum"=enum16{"Init", "Log", "Read"}."Log", "state Name"=w5192) -> ()  [unwired: 8 in, 2 out]
          }
          frame condition #1 {
          }
        }
        n2281 = call "progress string(SubVI).vi"("String 3"=w5158, "String in"=w5159) -> ("String out"=w5160:string)  [unwired: 9 in]
        n2282 = call "FGV Driver Data.vi"("DUT index(1-60)"=w5157) -> ("DUT SC"=w5156:bool)  [unwired: 7 in, 3 out]
        n2283 = case shown="False" w5156 {
          tunnel: [w5185 _] -> w5165
          tunnel: w5162 -> [w5184 _]
          frame False {
            w5172 = T11 {"command"="", "command data"=variant} ("element")
            w5171 = "MEAS.mux6_1"
            n2284 = To Variant(anything=T4."mux6-1_channel0" ("mux6_1(3wires)_encode")) -> (Variant=w5170:variant)
            n2285 = To Variant(anything=T4."mux6_1_channel6_3" ("mux6_1(3wires)_encode")) -> (Variant=w5182:variant)
            n2286 = To Variant(anything=T4."mux6_1_channel6_2" ("mux6_1(3wires)_encode")) -> (Variant=w5180:variant)
            n2287 = Bundle By Name(cluster=w5172, "command"=w5171, "command data"=w5180) -> (w5179:T11)
            n2288 = Bundle By Name(cluster=w5172, "command"=w5171, "command data"=w5182) -> (w5178:T11)
            n2289 = Bundle By Name(cluster=w5172, "command"=w5171, "command data"=w5170) -> ()  [unwired: 1 out]
            n2290 = Bundle By Name(cluster=w5172, "command"="MEAS.DMM dual read") -> (w5176:T11)
            n2291 = Build Array(w5179, w5178, w5176) -> (w5174:T11[])
            n2292 = Reverse 1D Array(array=w5174) -> (reversed array=w5175:T11[])
            n2293 = for {
              tunnel: [w5191] -> w5185 mode=indexing
              tunnel: w5184 -> [w5190]
              tunnel: w5175 -> [w5189] mode=indexing
              n2294 = Unbundle By Name(w5189) -> ("command"=w5188:string, "command data"=w5187:variant)
              n2295 = call "App enquece.vi"("Priority Enquece"=TRUE, "command data"=w5187, "command"=w5188, "queue in"=w5190) -> ("error out"=w5191:errorcluster)  [unwired: 6 in, 1 out]
            }
          }
          frame True {
          }
        }
        n2296 = Merge Errors(w5163, w5165) -> (w5164:errorcluster)
      }
      frame "Test DRV 49" {
        w5197 = 49  # DUT index(0-59)
        n2297 = disable-structure shown="LOGGING==TRUE" {
          disable-tunnel: w5199 -> [w5234 _]
          frame condition #0 (active) {
            n2298 = Empty String/Path?(string/path=w5234) -> (empty?=w5237:bool)
            n2299 = Select(t="Quece timeout", s=w5237, f=w5234) -> (s? t:f=w5233:string)
            n2300 = call "string log (SubVI).vi"("Enum"=enum16{"Init", "Log", "Read"}."Log", "state Name"=w5233) -> ()  [unwired: 8 in, 2 out]
          }
          frame condition #1 {
          }
        }
        n2301 = call "progress string(SubVI).vi"("String 3"=w5199, "String in"=w5200) -> ("String out"=w5201:string)  [unwired: 9 in]
        n2302 = call "FGV Driver Data.vi"("DUT index(1-60)"=w5197) -> ("DUT SC"=w5198:bool)  [unwired: 7 in, 3 out]
        n2303 = case shown="False" w5198 {
          tunnel: [w5226 _] -> w5206
          tunnel: w5203 -> [w5225 _]
          frame False {
            w5213 = T11 {"command"="", "command data"=variant} ("element")
            w5212 = "MEAS.mux6_1"
            n2304 = To Variant(anything=T4."mux6-1_channel0" ("mux6_1(3wires)_encode")) -> (Variant=w5211:variant)
            n2305 = To Variant(anything=T4."mux6_1_channel1_3" ("mux6_1(3wires)_encode")) -> (Variant=w5223:variant)
            n2306 = To Variant(anything=T4."mux6-1_channel1_2" ("mux6_1(3wires)_encode")) -> (Variant=w5221:variant)
            n2307 = Bundle By Name(cluster=w5213, "command"=w5212, "command data"=w5221) -> (w5220:T11)
            n2308 = Bundle By Name(cluster=w5213, "command"=w5212, "command data"=w5223) -> (w5219:T11)
            n2309 = Bundle By Name(cluster=w5213, "command"=w5212, "command data"=w5211) -> ()  [unwired: 1 out]
            n2310 = Bundle By Name(cluster=w5213, "command"="MEAS.DMM dual read") -> (w5217:T11)
            n2311 = Build Array(w5220, w5219, w5217) -> (w5215:T11[])
            n2312 = Reverse 1D Array(array=w5215) -> (reversed array=w5216:T11[])
            n2313 = for {
              tunnel: [w5232] -> w5226 mode=indexing
              tunnel: w5225 -> [w5231]
              tunnel: w5216 -> [w5230] mode=indexing
              n2314 = Unbundle By Name(w5230) -> ("command"=w5229:string, "command data"=w5228:variant)
              n2315 = call "App enquece.vi"("Priority Enquece"=TRUE, "command data"=w5228, "command"=w5229, "queue in"=w5231) -> ("error out"=w5232:errorcluster)  [unwired: 6 in, 1 out]
            }
          }
          frame True {
          }
        }
        n2316 = Merge Errors(w5204, w5206) -> (w5205:errorcluster)
      }
      frame "Test DRV 50" {
        w5238 = 50  # DUT index(0-59)
        n2317 = disable-structure shown="LOGGING==TRUE" {
          disable-tunnel: w5240 -> [w5275 _]
          frame condition #0 (active) {
            n2318 = Empty String/Path?(string/path=w5275) -> (empty?=w5278:bool)
            n2319 = Select(t="Quece timeout", s=w5278, f=w5275) -> (s? t:f=w5274:string)
            n2320 = call "string log (SubVI).vi"("Enum"=enum16{"Init", "Log", "Read"}."Log", "state Name"=w5274) -> ()  [unwired: 8 in, 2 out]
          }
          frame condition #1 {
          }
        }
        n2321 = call "progress string(SubVI).vi"("String 3"=w5240, "String in"=w5241) -> ("String out"=w5242:string)  [unwired: 9 in]
        n2322 = call "FGV Driver Data.vi"("DUT index(1-60)"=w5238) -> ("DUT SC"=w5239:bool)  [unwired: 7 in, 3 out]
        n2323 = case shown="False" w5239 {
          tunnel: [w5267 _] -> w5247
          tunnel: w5244 -> [w5266 _]
          frame False {
            w5254 = T11 {"command"="", "command data"=variant} ("element")
            w5253 = "MEAS.mux6_1"
            n2324 = To Variant(anything=T4."mux6-1_channel0" ("mux6_1(3wires)_encode")) -> (Variant=w5252:variant)
            n2325 = To Variant(anything=T4."mux6_1_channel2_3" ("mux6_1(3wires)_encode")) -> (Variant=w5264:variant)
            n2326 = To Variant(anything=T4."mux6_1_channel2_2" ("mux6_1(3wires)_encode")) -> (Variant=w5262:variant)
            n2327 = Bundle By Name(cluster=w5254, "command"=w5253, "command data"=w5262) -> (w5261:T11)
            n2328 = Bundle By Name(cluster=w5254, "command"=w5253, "command data"=w5264) -> (w5260:T11)
            n2329 = Bundle By Name(cluster=w5254, "command"=w5253, "command data"=w5252) -> ()  [unwired: 1 out]
            n2330 = Bundle By Name(cluster=w5254, "command"="MEAS.DMM dual read") -> (w5258:T11)
            n2331 = Build Array(w5261, w5260, w5258) -> (w5256:T11[])
            n2332 = Reverse 1D Array(array=w5256) -> (reversed array=w5257:T11[])
            n2333 = for {
              tunnel: [w5273] -> w5267 mode=indexing
              tunnel: w5266 -> [w5272]
              tunnel: w5257 -> [w5271] mode=indexing
              n2334 = Unbundle By Name(w5271) -> ("command"=w5270:string, "command data"=w5269:variant)
              n2335 = call "App enquece.vi"("Priority Enquece"=TRUE, "command data"=w5269, "command"=w5270, "queue in"=w5272) -> ("error out"=w5273:errorcluster)  [unwired: 6 in, 1 out]
            }
          }
          frame True {
          }
        }
        n2336 = Merge Errors(w5245, w5247) -> (w5246:errorcluster)
      }
      frame "Test DRV 51" {
        w5280 = 51  # DUT index(0-59)
        n2337 = disable-structure shown="LOGGING==TRUE" {
          disable-tunnel: w5281 -> [w5316 _]
          frame condition #0 (active) {
            n2338 = Empty String/Path?(string/path=w5316) -> (empty?=w5319:bool)
            n2339 = Select(t="Quece timeout", s=w5319, f=w5316) -> (s? t:f=w5315:string)
            n2340 = call "string log (SubVI).vi"("Enum"=enum16{"Init", "Log", "Read"}."Log", "state Name"=w5315) -> ()  [unwired: 8 in, 2 out]
          }
          frame condition #1 {
          }
        }
        n2341 = call "progress string(SubVI).vi"("String 3"=w5281, "String in"=w5282) -> ("String out"=w5283:string)  [unwired: 9 in]
        n2342 = call "FGV Driver Data.vi"("DUT index(1-60)"=w5280) -> ("DUT SC"=w5279:bool)  [unwired: 7 in, 3 out]
        n2343 = case shown="False" w5279 {
          tunnel: [w5308 _] -> w5288
          tunnel: w5285 -> [w5307 _]
          frame False {
            w5295 = T11 {"command"="", "command data"=variant} ("element")
            w5294 = "MEAS.mux6_1"
            n2344 = To Variant(anything=T4."mux6-1_channel0" ("mux6_1(3wires)_encode")) -> (Variant=w5293:variant)
            n2345 = To Variant(anything=T4."mux6_1_channel3_3" ("mux6_1(3wires)_encode")) -> (Variant=w5305:variant)
            n2346 = To Variant(anything=T4."mux6_1_channel3_2" ("mux6_1(3wires)_encode")) -> (Variant=w5303:variant)
            n2347 = Bundle By Name(cluster=w5295, "command"=w5294, "command data"=w5303) -> (w5302:T11)
            n2348 = Bundle By Name(cluster=w5295, "command"=w5294, "command data"=w5305) -> (w5301:T11)
            n2349 = Bundle By Name(cluster=w5295, "command"=w5294, "command data"=w5293) -> ()  [unwired: 1 out]
            n2350 = Bundle By Name(cluster=w5295, "command"="MEAS.DMM dual read") -> (w5299:T11)
            n2351 = Build Array(w5302, w5301, w5299) -> (w5297:T11[])
            n2352 = Reverse 1D Array(array=w5297) -> (reversed array=w5298:T11[])
            n2353 = for {
              tunnel: [w5314] -> w5308 mode=indexing
              tunnel: w5307 -> [w5313]
              tunnel: w5298 -> [w5312] mode=indexing
              n2354 = Unbundle By Name(w5312) -> ("command"=w5311:string, "command data"=w5310:variant)
              n2355 = call "App enquece.vi"("Priority Enquece"=TRUE, "command data"=w5310, "command"=w5311, "queue in"=w5313) -> ("error out"=w5314:errorcluster)  [unwired: 6 in, 1 out]
            }
          }
          frame True {
          }
        }
        n2356 = Merge Errors(w5286, w5288) -> (w5287:errorcluster)
      }
      frame "Test DRV 52" {
        w5321 = 52  # DUT index(0-59)
        n2357 = disable-structure shown="LOGGING==TRUE" {
          disable-tunnel: w5322 -> [w5357 _]
          frame condition #0 (active) {
            n2358 = Empty String/Path?(string/path=w5357) -> (empty?=w5360:bool)
            n2359 = Select(t="Quece timeout", s=w5360, f=w5357) -> (s? t:f=w5356:string)
            n2360 = call "string log (SubVI).vi"("Enum"=enum16{"Init", "Log", "Read"}."Log", "state Name"=w5356) -> ()  [unwired: 8 in, 2 out]
          }
          frame condition #1 {
          }
        }
        n2361 = call "progress string(SubVI).vi"("String 3"=w5322, "String in"=w5323) -> ("String out"=w5324:string)  [unwired: 9 in]
        n2362 = call "FGV Driver Data.vi"("DUT index(1-60)"=w5321) -> ("DUT SC"=w5320:bool)  [unwired: 7 in, 3 out]
        n2363 = case shown="False" w5320 {
          tunnel: [w5349 _] -> w5329
          tunnel: w5326 -> [w5348 _]
          frame False {
            w5336 = T11 {"command"="", "command data"=variant} ("element")
            w5335 = "MEAS.mux6_1"
            n2364 = To Variant(anything=T4."mux6-1_channel0" ("mux6_1(3wires)_encode")) -> (Variant=w5334:variant)
            n2365 = To Variant(anything=T4."mux6_1_channel4_3" ("mux6_1(3wires)_encode")) -> (Variant=w5346:variant)
            n2366 = To Variant(anything=T4."mux6_1_channel4_2" ("mux6_1(3wires)_encode")) -> (Variant=w5344:variant)
            n2367 = Bundle By Name(cluster=w5336, "command"=w5335, "command data"=w5344) -> (w5343:T11)
            n2368 = Bundle By Name(cluster=w5336, "command"=w5335, "command data"=w5346) -> (w5342:T11)
            n2369 = Bundle By Name(cluster=w5336, "command"=w5335, "command data"=w5334) -> ()  [unwired: 1 out]
            n2370 = Bundle By Name(cluster=w5336, "command"="MEAS.DMM dual read") -> (w5340:T11)
            n2371 = Build Array(w5343, w5342, w5340) -> (w5338:T11[])
            n2372 = Reverse 1D Array(array=w5338) -> (reversed array=w5339:T11[])
            n2373 = for {
              tunnel: [w5355] -> w5349 mode=indexing
              tunnel: w5348 -> [w5354]
              tunnel: w5339 -> [w5353] mode=indexing
              n2374 = Unbundle By Name(w5353) -> ("command"=w5352:string, "command data"=w5351:variant)
              n2375 = call "App enquece.vi"("Priority Enquece"=TRUE, "command data"=w5351, "command"=w5352, "queue in"=w5354) -> ("error out"=w5355:errorcluster)  [unwired: 6 in, 1 out]
            }
          }
          frame True {
          }
        }
        n2376 = Merge Errors(w5327, w5329) -> (w5328:errorcluster)
      }
      frame "Test DRV 53" {
        w5361 = 53  # DUT index(0-59)
        n2377 = disable-structure shown="LOGGING==TRUE" {
          disable-tunnel: w5363 -> [w5398 _]
          frame condition #0 (active) {
            n2378 = Empty String/Path?(string/path=w5398) -> (empty?=w5401:bool)
            n2379 = Select(t="Quece timeout", s=w5401, f=w5398) -> (s? t:f=w5397:string)
            n2380 = call "string log (SubVI).vi"("Enum"=enum16{"Init", "Log", "Read"}."Log", "state Name"=w5397) -> ()  [unwired: 8 in, 2 out]
          }
          frame condition #1 {
          }
        }
        n2381 = call "progress string(SubVI).vi"("String 3"=w5363, "String in"=w5364) -> ("String out"=w5365:string)  [unwired: 9 in]
        n2382 = call "FGV Driver Data.vi"("DUT index(1-60)"=w5361) -> ("DUT SC"=w5362:bool)  [unwired: 7 in, 3 out]
        n2383 = case shown="False" w5362 {
          tunnel: [w5390 _] -> w5370
          tunnel: w5367 -> [w5389 _]
          frame False {
            w5375 = T11 {"command"="", "command data"=variant} ("element")
            w5377 = "MEAS.mux6_1"
            n2384 = To Variant(anything=T4."mux6-1_channel0" ("mux6_1(3wires)_encode")) -> (Variant=w5376:variant)
            n2385 = To Variant(anything=T4."mux6_1_channel5_3" ("mux6_1(3wires)_encode")) -> (Variant=w5387:variant)
            n2386 = To Variant(anything=T4."mux6_1_channel5_2" ("mux6_1(3wires)_encode")) -> (Variant=w5385:variant)
            n2387 = Bundle By Name(cluster=w5375, "command"=w5377, "command data"=w5385) -> (w5384:T11)
            n2388 = Bundle By Name(cluster=w5375, "command"=w5377, "command data"=w5387) -> (w5383:T11)
            n2389 = Bundle By Name(cluster=w5375, "command"=w5377, "command data"=w5376) -> ()  [unwired: 1 out]
            n2390 = Bundle By Name(cluster=w5375, "command"="MEAS.DMM dual read") -> (w5381:T11)
            n2391 = Build Array(w5384, w5383, w5381) -> (w5379:T11[])
            n2392 = Reverse 1D Array(array=w5379) -> (reversed array=w5380:T11[])
            n2393 = for {
              tunnel: [w5396] -> w5390 mode=indexing
              tunnel: w5389 -> [w5395]
              tunnel: w5380 -> [w5394] mode=indexing
              n2394 = Unbundle By Name(w5394) -> ("command"=w5393:string, "command data"=w5392:variant)
              n2395 = call "App enquece.vi"("Priority Enquece"=TRUE, "command data"=w5392, "command"=w5393, "queue in"=w5395) -> ("error out"=w5396:errorcluster)  [unwired: 6 in, 1 out]
            }
          }
          frame True {
          }
        }
        n2396 = Merge Errors(w5368, w5370) -> (w5369:errorcluster)
      }
      frame "Test DRV 54" {
        w5403 = 54  # DUT index(0-59)
        n2397 = disable-structure shown="LOGGING==TRUE" {
          disable-tunnel: w5404 -> [w5439 _]
          frame condition #0 (active) {
            n2398 = Empty String/Path?(string/path=w5439) -> (empty?=w5442:bool)
            n2399 = Select(t="Quece timeout", s=w5442, f=w5439) -> (s? t:f=w5438:string)
            n2400 = call "string log (SubVI).vi"("Enum"=enum16{"Init", "Log", "Read"}."Log", "state Name"=w5438) -> ()  [unwired: 8 in, 2 out]
          }
          frame condition #1 {
          }
        }
        n2401 = call "progress string(SubVI).vi"("String 3"=w5404, "String in"=w5405) -> ("String out"=w5406:string)  [unwired: 9 in]
        n2402 = call "FGV Driver Data.vi"("DUT index(1-60)"=w5403) -> ("DUT SC"=w5402:bool)  [unwired: 7 in, 3 out]
        n2403 = case shown="False" w5402 {
          tunnel: [w5431 _] -> w5411
          tunnel: w5408 -> [w5430 _]
          frame False {
            w5418 = T11 {"command"="", "command data"=variant} ("element")
            w5417 = "MEAS.mux6_1"
            n2404 = To Variant(anything=T4."mux6-1_channel0" ("mux6_1(3wires)_encode")) -> (Variant=w5416:variant)
            n2405 = To Variant(anything=T4."mux6_1_channel6_3" ("mux6_1(3wires)_encode")) -> (Variant=w5428:variant)
            n2406 = To Variant(anything=T4."mux6_1_channel6_2" ("mux6_1(3wires)_encode")) -> (Variant=w5426:variant)
            n2407 = Bundle By Name(cluster=w5418, "command"=w5417, "command data"=w5426) -> (w5425:T11)
            n2408 = Bundle By Name(cluster=w5418, "command"=w5417, "command data"=w5428) -> (w5424:T11)
            n2409 = Bundle By Name(cluster=w5418, "command"=w5417, "command data"=w5416) -> ()  [unwired: 1 out]
            n2410 = Bundle By Name(cluster=w5418, "command"="MEAS.DMM dual read") -> (w5422:T11)
            n2411 = Build Array(w5425, w5424, w5422) -> (w5420:T11[])
            n2412 = Reverse 1D Array(array=w5420) -> (reversed array=w5421:T11[])
            n2413 = for {
              tunnel: [w5437] -> w5431 mode=indexing
              tunnel: w5430 -> [w5436]
              tunnel: w5421 -> [w5435] mode=indexing
              n2414 = Unbundle By Name(w5435) -> ("command"=w5434:string, "command data"=w5433:variant)
              n2415 = call "App enquece.vi"("Priority Enquece"=TRUE, "command data"=w5433, "command"=w5434, "queue in"=w5436) -> ("error out"=w5437:errorcluster)  [unwired: 6 in, 1 out]
            }
          }
          frame True {
          }
        }
        n2416 = Merge Errors(w5409, w5411) -> (w5410:errorcluster)
      }
